vi "Save to TDMS Core.vi"(8 "Error In":errorcluster, 10 "TDMS Ref":refnum<k34>, 11 "LHW-WfmBasicProperties in":refnum<class "LHW-WfmBasicProperties.lvclass">) -> (0 "Error Out":errorcluster, 3 "LHW-WfmBasicProperties out":refnum<class "LHW-WfmBasicProperties.lvclass">)   [LabVIEW 2014, in "LHW-Data.lvlib" / "LHW-WfmBasicProperties.lvclass"]
doc: "Save data to TDMS file."
uses:
  LHW-WfmBasicProperties.lvclass
  LHW-WfmBasicProperties.lvclass/LHW-WfmBasicProperties.ctl
  LHW-Data/LHW-Data.lvclass
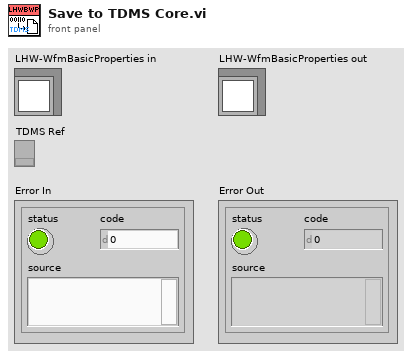
[diagram p1: front panel]
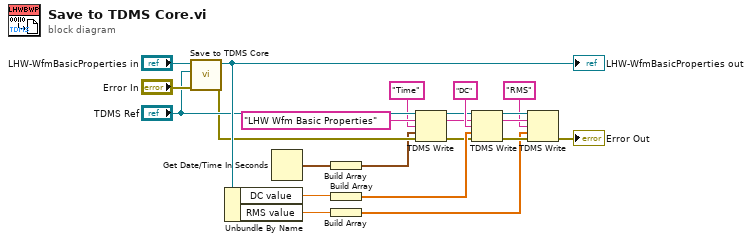
[diagram p0: block diagram]
diagram:
  n1 = call-parent "Save to TDMS Core.vi"("Error In"="Error In", "TDMS Ref"="TDMS Ref", "LHW-Data in"="LHW-WfmBasicProperties in") -> ("Error Out"=w5:errorcluster, "LHW-Data out"=w20:refnum<class "LHW-WfmBasicProperties.lvclass">)  [unwired: 7 in]
  "LHW-WfmBasicProperties out" <- w20
  n2 = Unbundle By Name(w20) -> ("DC value"=w19:dbl[unit], "RMS value"=w12:dbl[unit])
  n3 = Get Date/Time In Seconds() -> (seconds since 1Jan1904=w3:timestamp)
  n4 = Build Array(w3) -> (w1:timestamp[])
  n5 = Build Array(w19) -> (w18:dbl[unit][])
  n6 = Build Array(w12) -> (w11:dbl[unit][])
  n7 = TDMS Write(0:"TDMS Ref", 5:"LHW Wfm Basic Properties" ("group name in (Untitled)"), 7:"Time", 9:w1, 11:w5) -> (4:w9:refnum<k34>, 6:w8:string, 15:w7:errorcluster)  [unwired: 1 in, 1 out]
  n8 = TDMS Write(0:w9, 5:w8, 7:"DC", 9:w18, 11:w7) -> (4:w17:refnum<k34>, 6:w16:string, 15:w15:errorcluster)  [unwired: 1 in, 1 out]
  n9 = TDMS Write(0:w17, 5:w16, 7:"RMS", 9:w11, 11:w15) -> (15:→"Error Out":errorcluster)  [unwired: 1 in, 3 out]
